vi "Kernel - Error Handler.vi"(7 "data in - Error Handler":T1, 8 "error in":errorcluster, 10 "State":string, 11 "message queue":refnum<queue>) -> (0 "error out":errorcluster, 3 "message queue (out)":refnum<queue>, 4 "Stop?":bool, 5 "data out - Error Handler":T1)   [LabVIEW 2021]
uses:
  Typedefs/Data - Error Handler.ctl
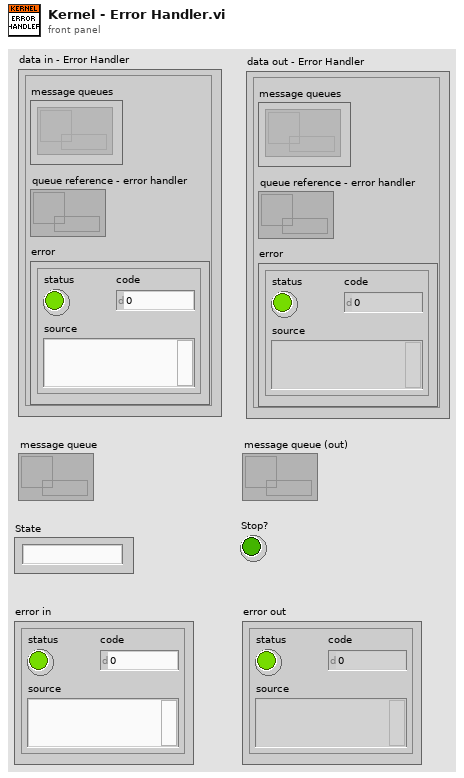
[diagram p1: front panel]
types:
  T1 = typedef "Data - Error Handler.ctl" = cluster{"message queues":refnum<queue>[], "queue reference - error handler":refnum<queue>, "error":errorcluster}
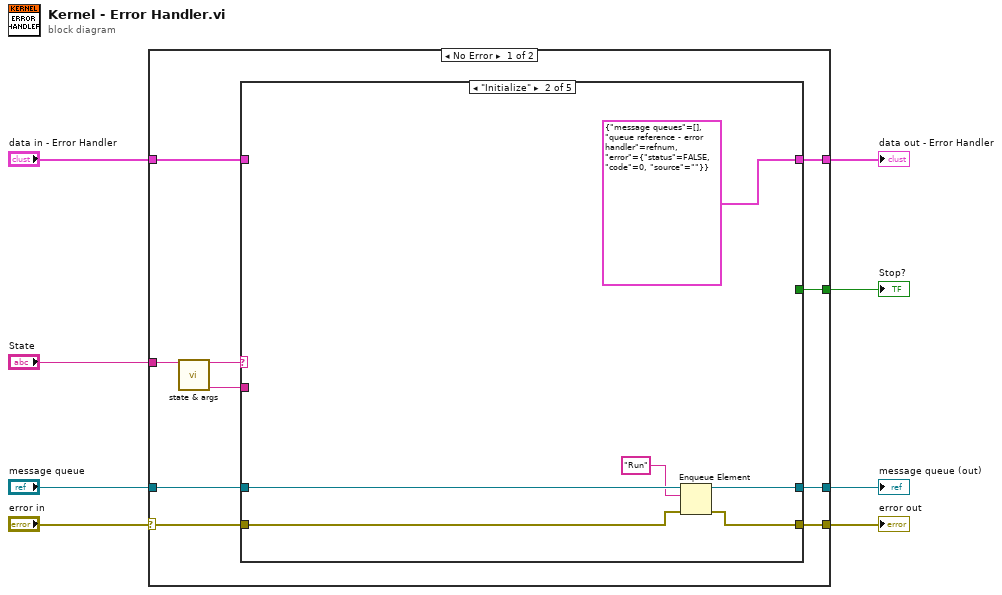
[diagram p0: block diagram]
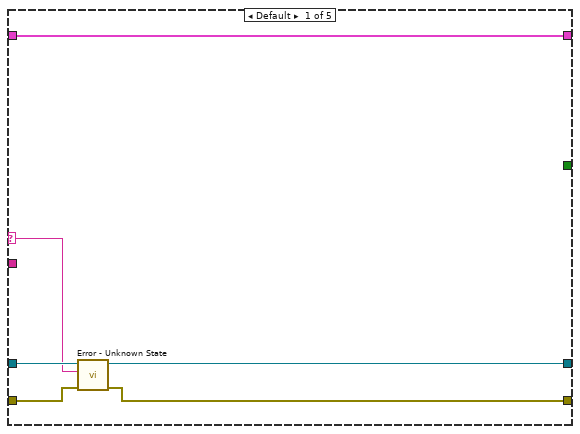
[diagram p2: hidden frame]
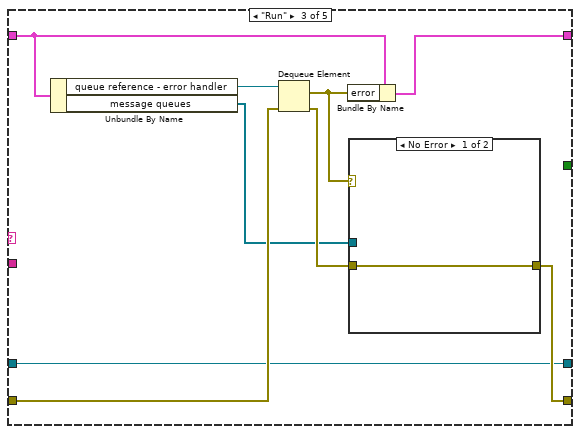
[diagram p3: hidden frame]
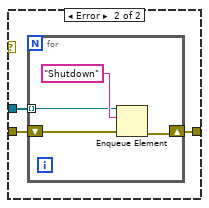
[diagram p4: hidden frame]
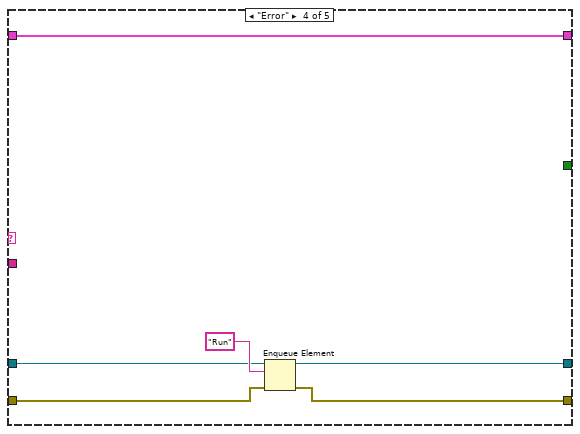
[diagram p5: hidden frame]
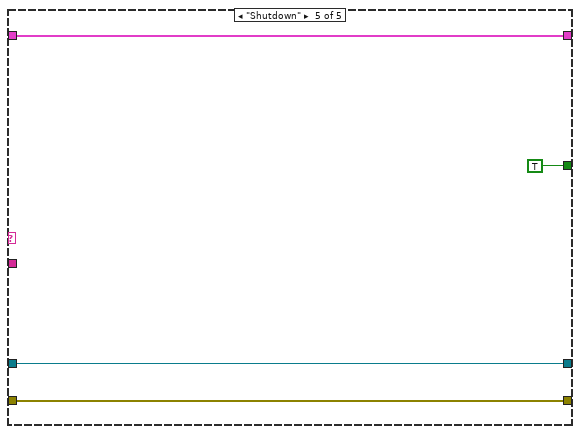
[diagram p6: hidden frame]
diagram:
  n1 = case shown="No Error" "error in" {
    selector: "error in" -> [w14 w58]
    tunnel: "State" -> [w18 _]
    tunnel: "message queue" -> [w15 w59]
    tunnel: "data in - Error Handler" -> [w13 w60]
    tunnel: [w12 w59] -> w4
    tunnel: [w11 w58] -> w3
    tunnel: [w10 w60] -> w2
    tunnel: [w9 _] -> w1
    frame No Error {
      n2 = call "state & args.vi"("state:args"=w18) -> ("args"=w16:string, "state"=w17:string)  [unwired: 9 in]
      n3 = case shown="\"Initialize\"" w17 {
        selector: w17 -> [w22 _ _ _ _]
        tunnel: w16 -> [_ _ _ _ _]
        tunnel: w15 -> [w24 w30 w31 w50 w56]
        tunnel: w14 -> [w23 w28 w38 w49 w55]
        tunnel: w13 -> [w19 _ w37 w53 w54]
        tunnel: [w21 w29 w31 w51 w56] -> w12
        tunnel: [w20 w27 w32 w48 w55] -> w11
        tunnel: [w19 T1 {"message queues"=[], "queue reference - error handler"=refnum, "error"={"status"=FALSE, "code"=0, "source"=""}} ("data in - Error Handler") w36 w53 w54] -> w10
        tunnel: [_ _ _ _ TRUE] -> w9
        frame Default {
          n4 = call "Error - Unknown State.vi"("error in"=w23, "state"=w22, "queue"=w24) -> ("error out"=w20:errorcluster, "queue out"=w21:refnum<queue>)  [unwired: 7 in]
        }
        frame "Initialize" {
          n5 = Enqueue Element(queue=w30, element="Run", error in (no error)=w28) -> (queue out=w29:refnum<queue>, error out=w27:errorcluster)  [unwired: 1 in, 1 out]
        }
        frame "Run" {
          n6 = Unbundle By Name(w37) -> ("queue reference - error handler"=w39:refnum<queue>, "message queues"=w33:refnum<queue>[])
          n7 = Dequeue Element(queue=w39, error in (no error)=w38) -> (element=w35:errorcluster, error out=w34:errorcluster)  [unwired: 1 in, 2 out]
          n8 = Bundle By Name(cluster=w37, "error"=w35) -> (w36:T1)
          n9 = case shown="No Error" w35 {
            tunnel: w34 -> [w40 w43]
            tunnel: w33 -> [_ w41]
            tunnel: [w40 w42] -> w32
            frame No Error {
            }
            frame Error {
              n10 = for {
                shift-right: [w46] -> w42
                shift-left: w43 -> [w47]
                tunnel: w41 -> [w44] mode=indexing
                n11 = Enqueue Element(queue=w44, element="Shutdown", error in (no error)=w47) -> (error out=w46:errorcluster)  [unwired: 1 in, 2 out]
              }
            }
          }
        }
        frame "Error" {
          n12 = Enqueue Element(queue=w50, element="Run", error in (no error)=w49) -> (queue out=w51:refnum<queue>, error out=w48:errorcluster)  [unwired: 1 in, 1 out]
        }
        frame "Shutdown" {
        }
      }
    }
    frame Error {
    }
  }
  "error out" <- w3
  "Stop?" <- w1
  "message queue (out)" <- w4
  "data out - Error Handler" <- w2
